vi "Close.vi"(8 "error in (no error)":errorcluster, 11 "dotNET TCP Socket in":refnum<class "dotNET TCP Socket.lvclass">) -> (0 "error out":errorcluster)   [LabVIEW 2013, in "dotNET SSL Socket.lvlib" / "dotNET TCP Socket.lvclass"]
doc: "Closes the socket connection."
uses:
  dotNET TCP Socket.lvclass
  dotNET TCP Socket.lvclass/dotNET TCP Socket.ctl
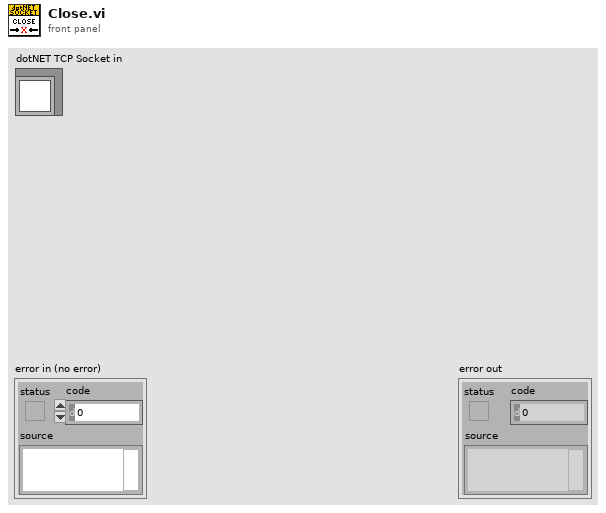
[diagram p1: front panel]
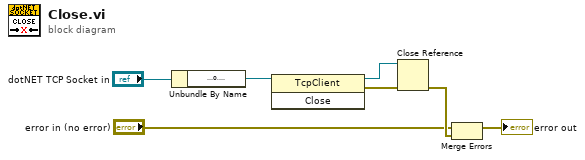
[diagram p0: block diagram]
diagram:
  n1 = Unbundle By Name("dotNET TCP Socket in") -> ("TcpClient"=w6:refnum<k24>)
  n2 = invoke class="TcpClient" method="Close"(reference=w6) -> (reference out=w4:refnum<k24>, error out=w5:errorcluster)  [unwired: 2 in, 1 out]
  n3 = Close Reference(reference=w4, error in (no error)=w5) -> (error out=w3:errorcluster)
  n4 = Merge Errors("error in (no error)", w3) -> (→"error out":errorcluster)
